vi "Manual Test.vi"() -> ()   [LabVIEW 2018, in "Omega Platinum Series.lvlib"]
uses:
  <instrlib>/Omega Platinum Series/Omega Platinum Series.lvlib
  <instrlib>/Omega Platinum Series/Public/Type Defs/Filter Constant.ctl
  <instrlib>/Omega Platinum Series/Public/Type Defs/Setpoint Type.ctl
  <instrlib>/Omega Platinum Series/Public/Type Defs/Display Temperature Units.ctl
  <instrlib>/Omega Platinum Series/Public/Type Defs/System State.ctl
panel:
  in  "Change Retry Attempts":bool
  in  "Retry Attempts (0)":i32 min=0
  in  "Get Current System State Btn":bool
  out "Current System State":T1
  out "Running":bool
  in  "Start/Stop Btn":bool
  out "Status Setpoint 2 Type":T2=enum."Deviation"
  in  "Change Address Btn":bool
  in  "Initialize Resource Btn":bool
  out "Status Serial Address (hex)":i32 format="%x"
  in  "Get Serial Address Btns":bool
  in  "Get Current Temperature Btn":bool
  out "Current Temperature Reading":string
  in  "Configure Temperature Units":T3
  in  "Set Temperature Units Btn":bool
  in  "Get Temperature Units Btn":bool
  out "Status Temperature Units":string
  in  "Setpoint 2 Type":T2=enum."Deviation"
  in  "Get Setpoint 2 Btn":bool
  in  "Set Setpoint 2 Btn":bool
  out "Status Setpoint 2":dbl
  in  "Configure Setpoint 2":dbl
  in  "Get Setpoint 1 Btn":bool
  in  "Set Setpoint 1 Btn":bool
  out "Status Setpoint 1":dbl
  in  "Configure Setpoint 1":dbl
  in  "Get Filter Constant Btn":bool
  out "Status Filter Constant":T4
  in  "Configure Filter Constant Btn":bool
  in  "Unit ID (-1, 0-199)":i32
  in  "Configure Filter Constant":T4
  out "error out":errorcluster
  in  "stop":bool
  in  "error in (no error)":errorcluster
  in  "Get Firmware Version Btn":bool
  out "Firmware Version":string
  in  "VISA resource name":refnum<visa-resource-name>
  # "Omega Platinum Series"
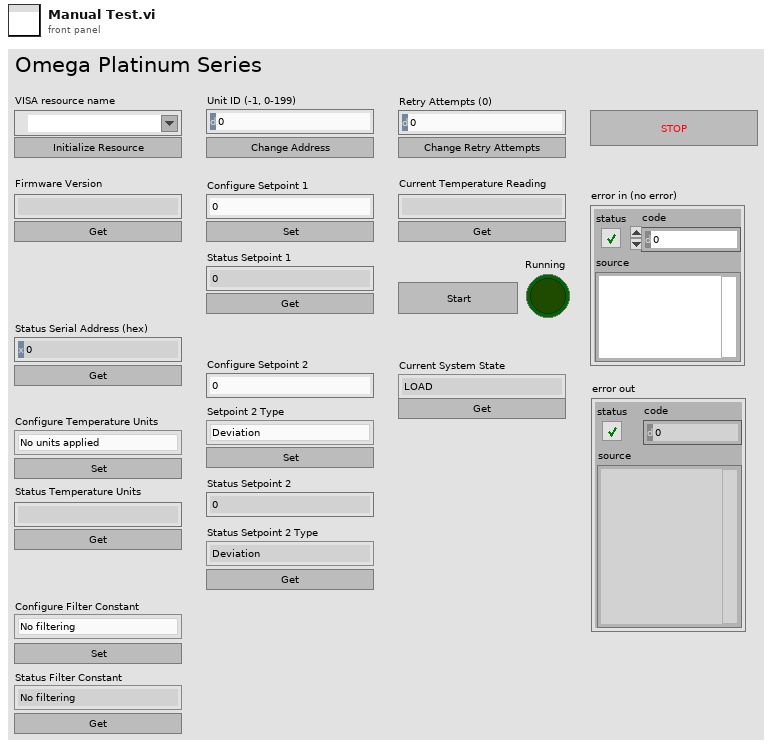
[diagram p1: front panel]
types:
  T1 = typedef "Omega Platinum Series.lvlib/System State.ctl" = enum16{"LOAD", "IDLE", "INPUT_ADJUST", "CONTROL_ADJUST", "MODIFY", "WAIT", "RUN", "STANDBY", "STOP", "PAUSE", "FAULT", "SHUTDOWN", "AUTOTUNE"}
  T2 = typedef "Omega Platinum Series.lvlib/Setpoint Type.ctl" = enum16{"Fixed Constant", "Deviation"}
  T3 = typedef "Omega Platinum Series.lvlib/Display Temperature Units.ctl" = enum16{"No units applied", "Celsius", "Fahrenheit"}
  T4 = typedef "Omega Platinum Series.lvlib/Filter Constant.ctl" = enum16{"No filtering", "X 2 filtering", "X 4 filtering", "X 8 filtering", "X 16 filtering", "X 32 filtering", "X 64 filtering", "X 128 filtering"}
  T5 = cluster{"Baud Rate":u32, "Parity":u16, "Flow Control":u16, "Data Bits":u16, "Stop Bits":u16}
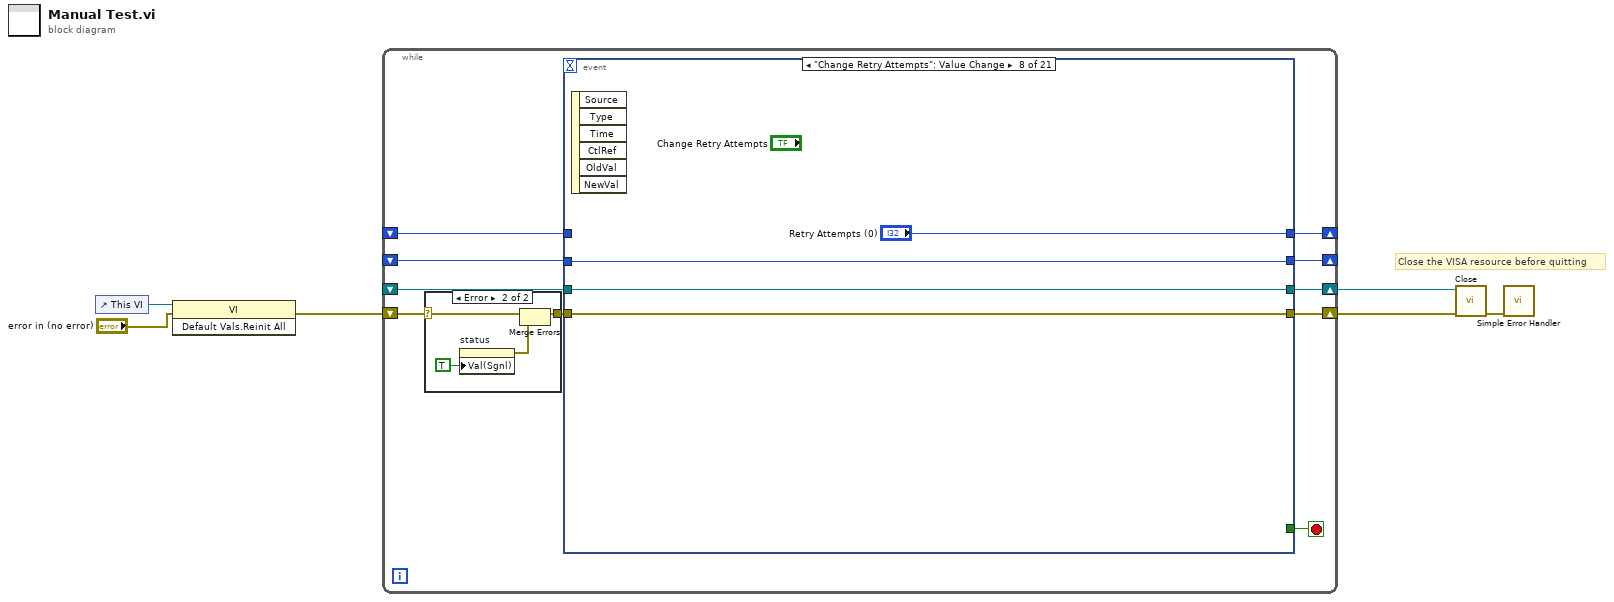
[diagram p0: block diagram]
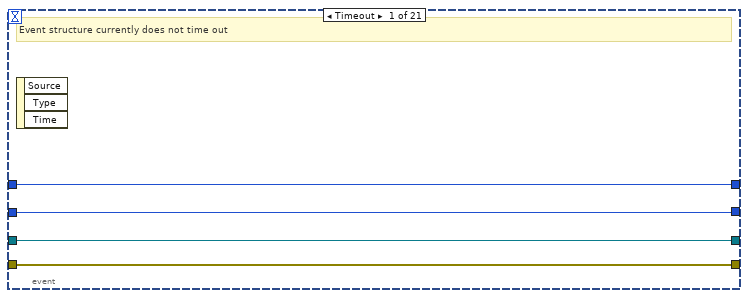
[diagram p3: hidden frame]
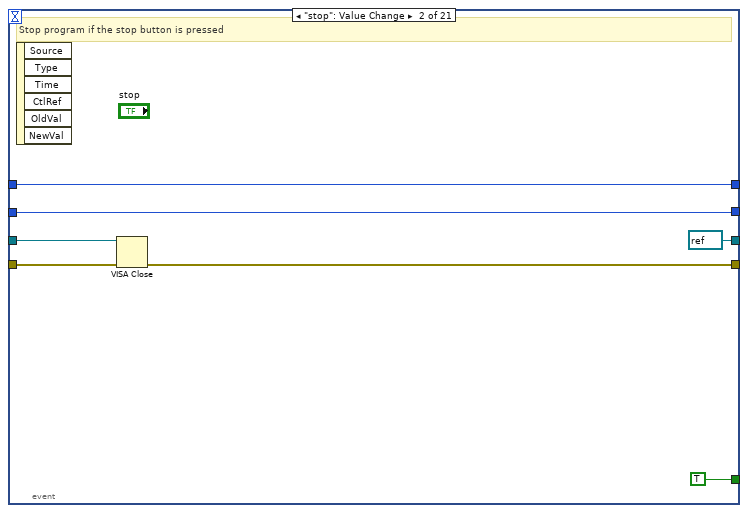
[diagram p4: hidden frame]
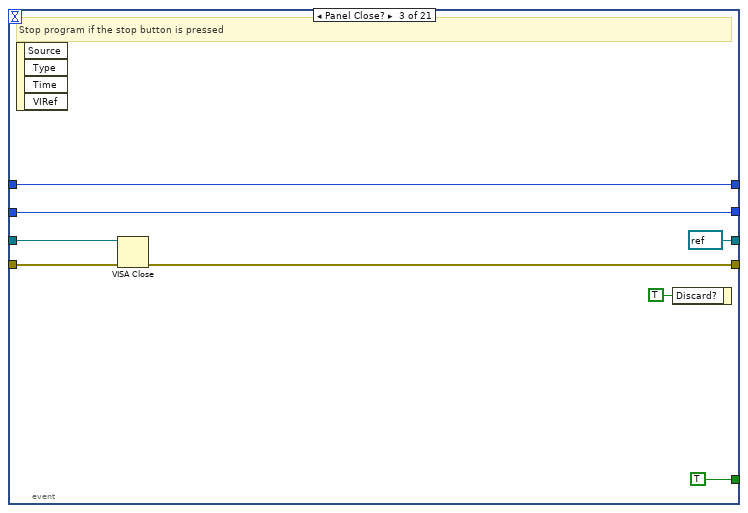
[diagram p5: hidden frame]
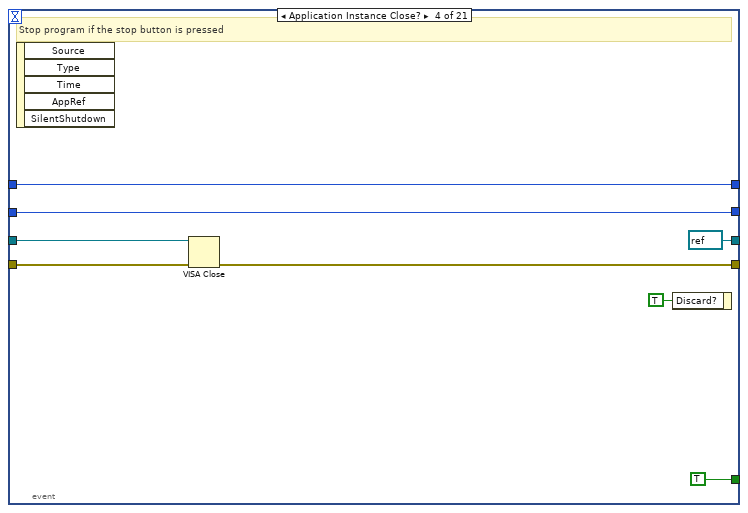
[diagram p6: hidden frame]
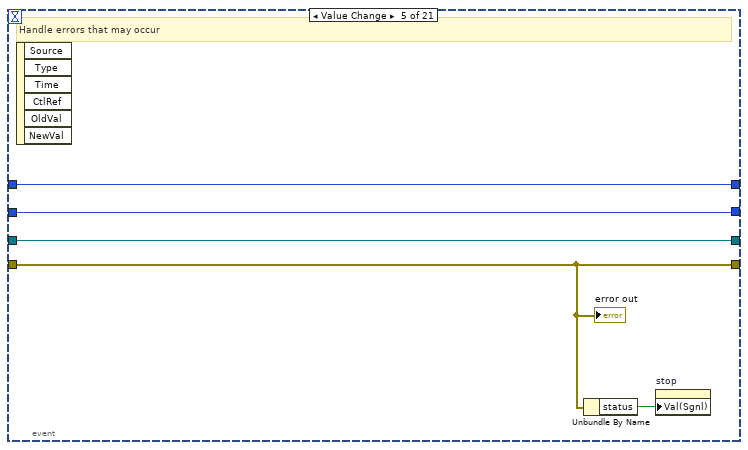
[diagram p7: hidden frame]
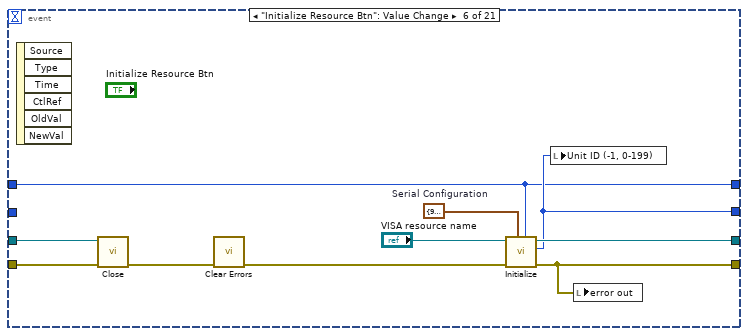
[diagram p8: hidden frame]
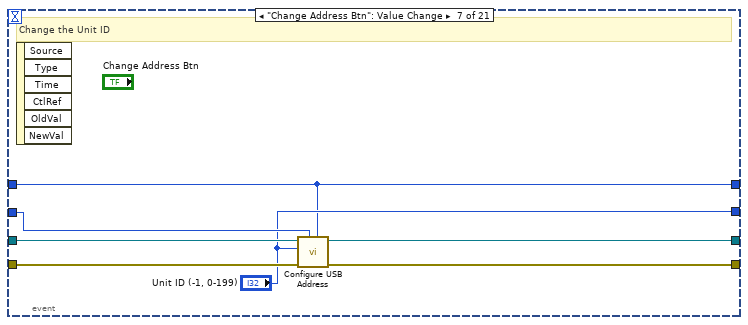
[diagram p9: hidden frame]
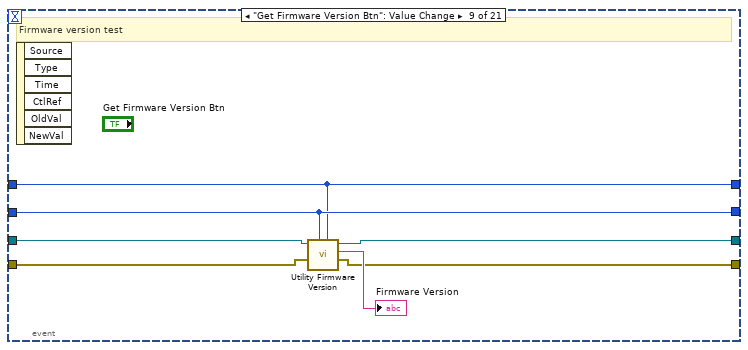
[diagram p10: hidden frame]
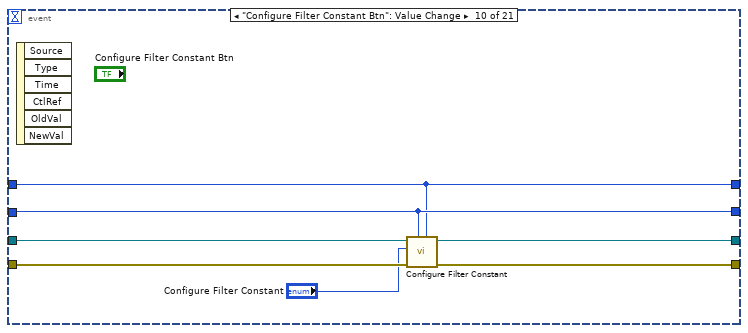
[diagram p11: hidden frame]
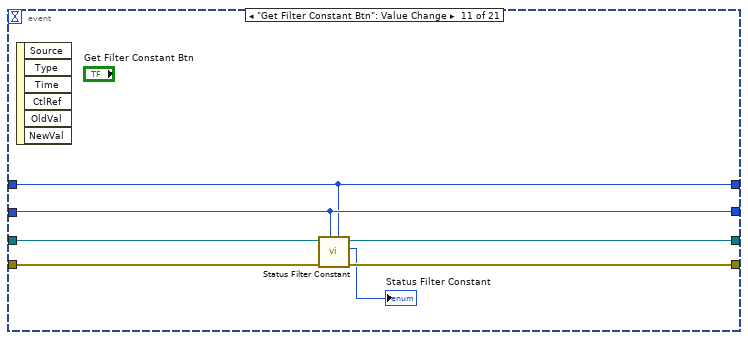
[diagram p12: hidden frame]
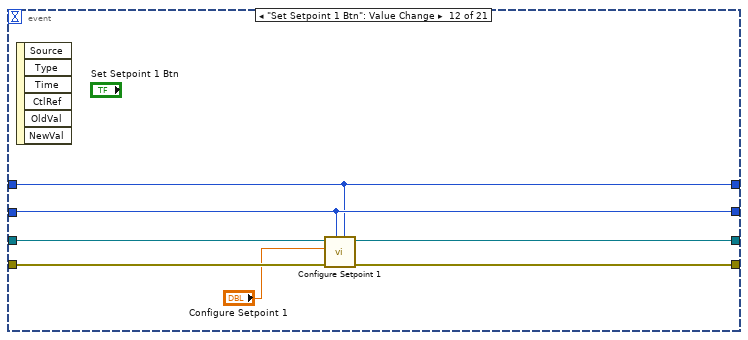
[diagram p13: hidden frame]
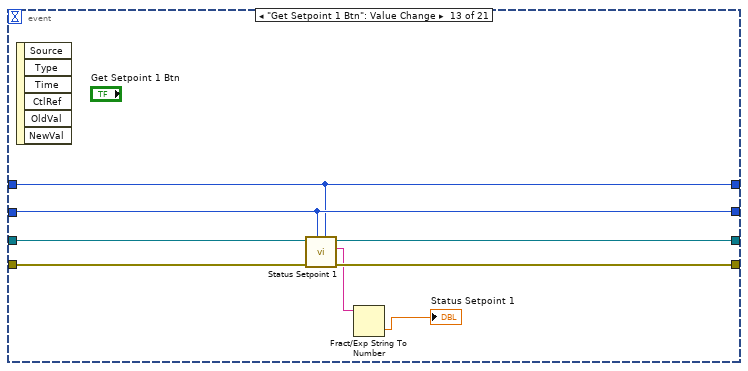
[diagram p14: hidden frame]
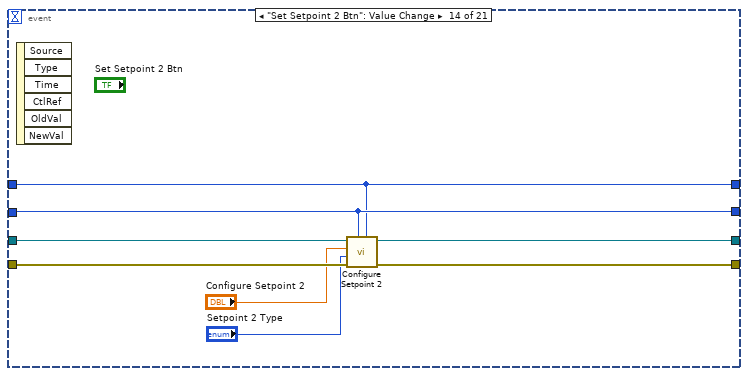
[diagram p15: hidden frame]
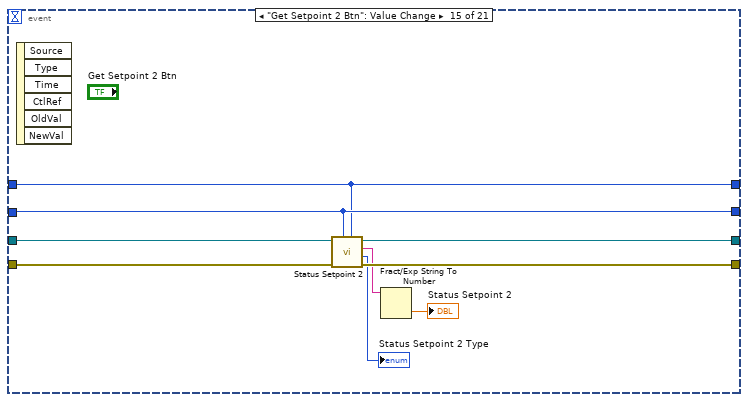
[diagram p16: hidden frame]
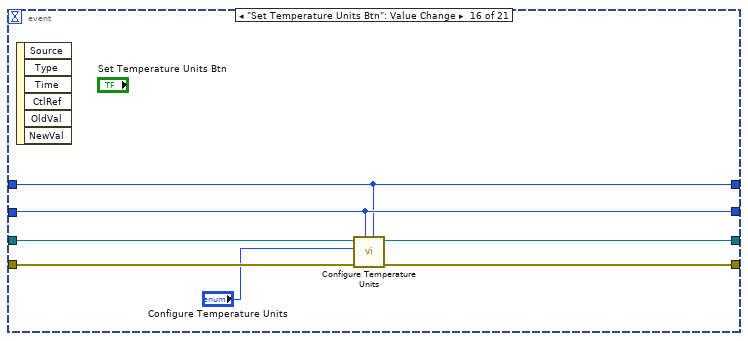
[diagram p17: hidden frame]
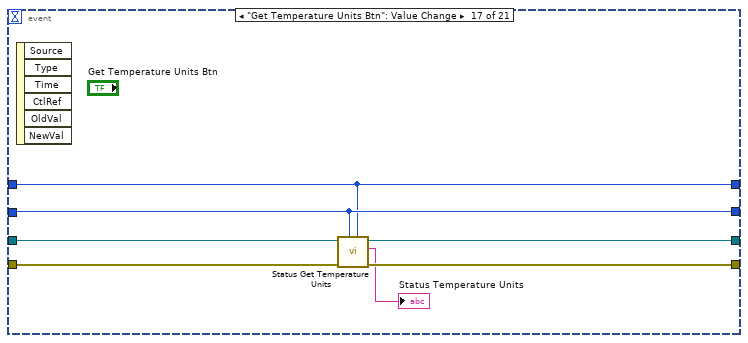
[diagram p18: hidden frame]
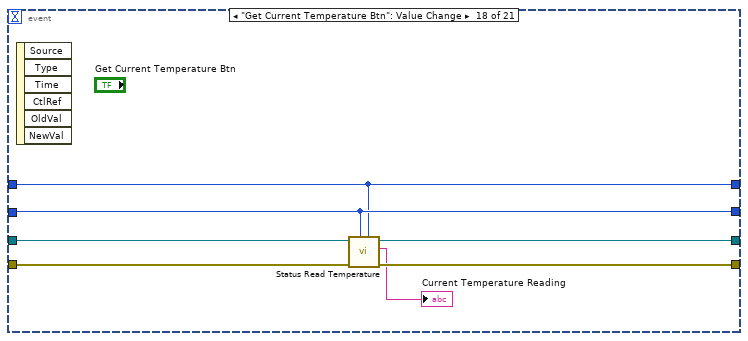
[diagram p19: hidden frame]
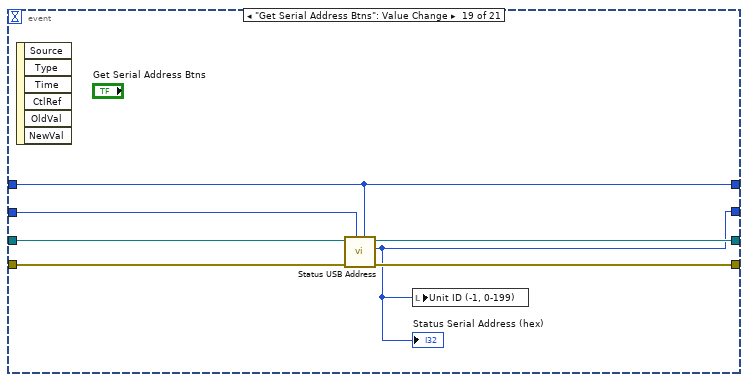
[diagram p20: hidden frame]
diagram:
  # "Close the VISA resource before quitting"
  n1 = control-ref of="This VI"() -> (w4:refnum<vi>)
  n2 = invoke class="VI" method="Default Vals.Reinit All"(reference=w4, error in="error in (no error)") -> (error out=w2:errorcluster)  [unwired: 1 in, 2 out]
  n3 = while {
    shift-right: [w13] -> w5
    shift-left: w2 -> [w12]
    shift-right: [w15] -> w6
    shift-left: _ -> [w16]
    shift-right: [w9] -> _
    shift-left: _ -> [w10]
    shift-right: [w7] -> _
    shift-left: _ -> [w8]
    stop <- w14 stop-if-true
    # "Manual Testing Finite State Machine"
    n4 = case shown="Error" w12 {
      selector: w12 -> [w17 w21]
      tunnel: [w17 w19] -> w11
      frame No Error {
      }
      frame Error {
        n5 = property on="status" class="Bool (strict)"("Val(Sgnl)"=TRUE ("Value (Signaling)")) -> (error out=w18:errorcluster)  [unwired: 2 in, 1 out]
        n6 = Merge Errors(w21, w18) -> (w19:errorcluster)
      }
    }
    n7 = event shown="[7] \"Change Retry Attempts\": Value Change" {
      selector: _ -> [_ _ _ _ _ _ _ _ _ _ _ _ _ _ _ _ _ _ _ _ _]
      dyn-events: _ -> [_ _ _ _ _ _ _ _ _ _ _ _ _ _ _ _ _ _ _ _ _]
      timeout: _ -> [_ _ _ _ _ _ _ _ _ _ _ _ _ _ _ _ _ _ _ _ _]
      tunnel: w16 -> [w25 w31 w35 w43 w53 w58 w70 w72 w80 w88 w94 w101 w109 w117 w126 w133 w140 w147 w155 w162 w183]
      tunnel: [w25 refnum<visa-resource-name> refnum ("VISA resource name (out)") refnum<visa-resource-name> refnum ("VISA resource name (out)") refnum<visa-resource-name> refnum ("VISA resource name (out)") w53 w61 w69 w72 w79 w86 w93 w100 w108 w116 w125 w132 w139 w146 w154 w160 w179] -> w15
      tunnel: w11 -> [w24 w29 w39 w47 w52 w62 w68 w71 w78 w87 w95 w102 w110 w118 w127 w134 w141 w148 w153 w161 w182]
      tunnel: [w24 w28 w36 w44 w52 w57 w67 w71 w77 w85 w92 w99 w107 w115 w124 w131 w138 w145 w152 w159 w181] -> w13
      tunnel: [_ TRUE TRUE TRUE _ _ _ _ _ _ _ _ _ _ _ _ _ _ _ _ _] -> w14
      tunnel: w10 -> [w23 w30 w38 w46 w51 _ w66 w73 w76 w84 w90 w98 w104 w112 w122 w129 w136 w143 w151 w163 w180]
      tunnel: [w23 w30 w38 w46 w51 w56 "Unit ID (-1, 0-199)" w73 w76 w84 w90 w98 w104 w112 w122 w129 w136 w143 w150 w158 w180] -> w9
      tunnel: w8 -> [w22 w26 w33 w41 w49 w54 w64 _ w75 w82 w89 w96 w103 w111 w119 w128 w135 w142 w149 w157 w178]
      tunnel: [w22 w26 w33 w41 w49 w54 w64 "Retry Attempts (0)" w75 w82 w89 w96 w103 w111 w119 w128 w135 w142 w149 w156 w178] -> w7
      event Timeout {
        # "Event structure currently does not time out"
        n8 = event-data() -> ()  [unwired: 1 in, 3 out]
      }
      event "stop": Value Change {
        # "Stop program if the stop button is pressed"
        n9 = event-data() -> ()  [unwired: 1 in, 6 out]
        n10 = VISA Close(VISA resource name=w31, error in (no error)=w29) -> (error out=w28:errorcluster)
      }
      event Panel Close? {
        # "Stop program if the stop button is pressed"
        n11 = event-data() -> ()  [unwired: 1 in, 4 out]
        n12 = VISA Close(VISA resource name=w35, error in (no error)=w39) -> (error out=w36:errorcluster)
        n13 = event-data("Discard?"=TRUE) -> ()  [unwired: 1 in, 1 out]
      }
      event Application Instance Close? {
        # "Stop program if the stop button is pressed"
        n14 = event-data() -> ()  [unwired: 1 in, 5 out]
        n15 = VISA Close(VISA resource name=w43, error in (no error)=w47) -> (error out=w44:errorcluster)
        n16 = event-data("Discard?"=TRUE) -> ()  [unwired: 1 in, 1 out]
      }
      event "error out.status": Value Change {
        # "Handle errors that may occur"
        n17 = event-data() -> ()  [unwired: 1 in, 6 out]
        n18 = Unbundle By Name(w52) -> ("status"=w50:bool)
        n19 = property on="stop" class="Bool (strict)"("Val(Sgnl)"=w50) -> ()  [unwired: 2 in, 2 out]
        "error out" <- w52
      }
      event "Initialize Resource Btn": Value Change {
        w63 = T5 {"Baud Rate"=9600, "Parity"=0, "Flow Control"=0, "Data Bits"=8, "Stop Bits"=10}  # Serial Configuration
        n20 = event-data() -> ()  [unwired: 1 in, 6 out]
        n21 = call <instrlib>:"Close.vi"("error in (no error)"=w62, "VISA resource name"=w58) -> ("error out"=w59:errorcluster)  [unwired: 9 in]
        n22 = call <vilib>:"Clear Errors.vi"("error in (no error)"=w59) -> ("error out"=w55:errorcluster)  [unwired: 5 in, 1 out]
        n23 = call <instrlib>:"Initialize.vi"("Retry Attempts (0)"=w54, "Serial Configuration"=w63, "error in (no error)"=w55, "VISA resource name"="VISA resource name") -> ("error out"=w57:errorcluster, "Address ID (-1 if ID Query = False)"=w56:i32, "VISA resource name out"=w61:refnum<visa-resource-name>)  [unwired: 5 in]
        n24 = local write "Unit ID (-1, 0-199)"(w56) -> ()
        n25 = local write "error out"(w57) -> ()
      }
      event "Change Address Btn": Value Change {
        # "Change the Unit ID"
        n26 = event-data() -> ()  [unwired: 1 in, 6 out]
        n27 = call <instrlib>:"Configure USB Address.vi"("Retry Attempts (0)"=w64, "Current Address (-1)"=w66, "error in (no error)"=w68, "New Address"="Unit ID (-1, 0-199)", "VISA resource name (in)"=w70) -> ("error out"=w67:errorcluster, "VISA resource name (out)"=w69:refnum<visa-resource-name>)  [unwired: 4 in, 1 out]
      }
      event "Change Retry Attempts": Value Change {
        n28 = event-data() -> ()  [unwired: 1 in, 6 out]
      }
      event "Get Firmware Version Btn": Value Change {
        # "Firmware version test"
        n29 = event-data() -> ()  [unwired: 1 in, 6 out]
        n30 = call <instrlib>:"Utility Firmware Version.vi"("Retry Attempts (0)"=w75, "Unit ID (-1)"=w76, "error in"=w78, "VISA resource name"=w80) -> ("error out"=w77:errorcluster, "Firmware Version"=→"Firmware Version":string, "VISA resource name out"=w79:refnum<visa-resource-name>)  [unwired: 5 in]
      }
      event "Configure Filter Constant Btn": Value Change {
        n31 = event-data() -> ()  [unwired: 1 in, 6 out]
        n32 = call <instrlib>:"Configure Filter Constant.vi"("Retry Attempts (0)"=w82, "Unit Address (-1)"=w84, "error in (no error)"=w87, "Filter Constant"="Configure Filter Constant", "VISA resource name (in)"=w88) -> ("error out"=w85:errorcluster, "VISA resource name (out)"=w86:refnum<visa-resource-name>)  [unwired: 4 in, 1 out]
      }
      event "Get Filter Constant Btn": Value Change {
        n33 = event-data() -> ()  [unwired: 1 in, 6 out]
        n34 = call <instrlib>:"Status Filter Constant.vi"("Retry Attempts (0)"=w89, "Unit Address (-1)"=w90, "error in (no error)"=w95, "VISA resource name (in)"=w94) -> ("error out"=w92:errorcluster, "Filter Constant"=→"Status Filter Constant":T4, "VISA resource name (out)"=w93:refnum<visa-resource-name>)  [unwired: 5 in]
      }
      event "Set Setpoint 1 Btn": Value Change {
        n35 = event-data() -> ()  [unwired: 1 in, 6 out]
        n36 = call <instrlib>:"Configure Setpoint 1.vi"("Retry Attempts (0)"=w96, "Unit Address (-1)"=w98, "error in (no error)"=w102, "Setpoint value"="Configure Setpoint 1", "VISA resource name (in)"=w101) -> ("error out"=w99:errorcluster, "VISA resource name (out)"=w100:refnum<visa-resource-name>)  [unwired: 4 in, 1 out]
      }
      event "Get Setpoint 1 Btn": Value Change {
        n37 = event-data() -> ()  [unwired: 1 in, 6 out]
        n38 = call <instrlib>:"Status Setpoint 1.vi"("Retry Attempts (0)"=w103, "Unit Address (-1)"=w104, "error in (no error)"=w110, "VISA resource name (in)"=w109) -> ("error out"=w107:errorcluster, "Setpoint 1"=w106:string, "VISA resource name (out)"=w108:refnum<visa-resource-name>)  [unwired: 5 in]
        n39 = Fract/Exp String To Number(string=w106) -> (number=→"Status Setpoint 1":dbl)  [unwired: 3 in, 1 out]
      }
      event "Set Setpoint 2 Btn": Value Change {
        n40 = event-data() -> ()  [unwired: 1 in, 6 out]
        n41 = call <instrlib>:"Configure Setpoint 2.vi"("Retry Attempts (0)"=w111, "Unit Address (-1)"=w112, "error in (no error)"=w118, "Setpoint Type (deviation)"="Setpoint 2 Type", "Setpoint value"="Configure Setpoint 2", "VISA resource name (in)"=w117) -> ("error out"=w115:errorcluster, "VISA resource name (out)"=w116:refnum<visa-resource-name>)  [unwired: 3 in, 1 out]
      }
      event "Get Setpoint 2 Btn": Value Change {
        n42 = event-data() -> ()  [unwired: 1 in, 6 out]
        n43 = call <instrlib>:"Status Setpoint 2.vi"("Retry Attempts (0)"=w119, "Unit Address (-1)"=w122, "error in (no error)"=w127, "VISA resource name (in)"=w126) -> ("error out"=w124:errorcluster, "Setpoint Type"=→"Status Setpoint 2 Type":T2, "Setpoint 2"=w121:string, "VISA resource name (out)"=w125:refnum<visa-resource-name>)  [unwired: 4 in]
        n44 = Fract/Exp String To Number(string=w121) -> (number=→"Status Setpoint 2":dbl)  [unwired: 3 in, 1 out]
      }
      event "Set Temperature Units Btn": Value Change {
        n45 = event-data() -> ()  [unwired: 1 in, 6 out]
        n46 = call <instrlib>:"Configure Temperature Units.vi"("Retry Attempts (0)"=w128, "Unit Address (-1)"=w129, "error in (no error)"=w134, "Temperature Units (Celsius)"="Configure Temperature Units", "VISA resource name (in)"=w133) -> ("error out"=w131:errorcluster, "VISA resource name (out)"=w132:refnum<visa-resource-name>)  [unwired: 4 in, 1 out]
      }
      event "Get Temperature Units Btn": Value Change {
        n47 = event-data() -> ()  [unwired: 1 in, 6 out]
        n48 = call <instrlib>:"Status Get Temperature Units.vi"("Retry Attempts (0)"=w135, "Unit Address (-1)"=w136, "error in (no error)"=w141, "VISA resource name (in)"=w140) -> ("error out"=w138:errorcluster, "Temperature Units"=→"Status Temperature Units":string, "VISA resource name (out)"=w139:refnum<visa-resource-name>)  [unwired: 5 in]
      }
      event "Get Current Temperature Btn": Value Change {
        n49 = event-data() -> ()  [unwired: 1 in, 6 out]
        n50 = call <instrlib>:"Status Read Temperature.vi"("Retry Attempts (0)"=w142, "Unit Address (-1)"=w143, "error in (no error)"=w148, "VISA resource name (in)"=w147) -> ("error out"=w145:errorcluster, "Temperature"=→"Current Temperature Reading":string, "VISA resource name (out)"=w146:refnum<visa-resource-name>)  [unwired: 5 in]
      }
      event "Get Serial Address Btns": Value Change {
        n51 = event-data() -> ()  [unwired: 1 in, 6 out]
        n52 = call <instrlib>:"Status USB Address.vi"("Retry Attempts (0)"=w149, "Unit Address (-1)"=w151, "error in (no error)"=w153, "VISA resource name (in)"=w155) -> ("error out"=w152:errorcluster, "Address"=w150:i32, "VISA resource name (out)"=w154:refnum<visa-resource-name>)  [unwired: 5 in]
        "Status Serial Address (hex)" <- w150
        n53 = local write "Unit ID (-1, 0-199)"(w150) -> ()
      }
      event "Start/Stop Btn": Value Change {
        n54 = event-data() -> ("NewVal"=→"Running":bool)  [unwired: 1 in, 5 out]
        n55 = case shown="True" "Start/Stop Btn" {
          tunnel: w163 -> [w167 w173]
          tunnel: w162 -> [w171 w177]
          tunnel: w161 -> [w169 w175]
          tunnel: [w170 w176] -> w160
          tunnel: [w168 w174] -> w159
          tunnel: [w167 w173] -> w158
          tunnel: w157 -> [w166 w172]
          tunnel: [w166 w172] -> w156
          frame False {
            # "Stop the controller."
            n56 = call <instrlib>:"Action Stop.vi"("Retry Attempts (0)"=w166, "Unit Address (-1)"=w167, "error in (no error)"=w169, "VISA resource name (in)"=w171) -> ("error out"=w168:errorcluster, "VISA resource name (out)"=w170:refnum<visa-resource-name>)  [unwired: 5 in, 1 out]
          }
          frame True {
            # "Start the controller."
            n57 = call <instrlib>:"Action Run.vi"("Retry Attempts (0)"=w172, "Unit Address (-1)"=w173, "error in (no error)"=w175, "VISA resource name (in)"=w177) -> ("error out"=w174:errorcluster, "VISA resource name (out)"=w176:refnum<visa-resource-name>)  [unwired: 5 in, 1 out]
          }
        }
      }
      event "Get Current System State Btn": Value Change {
        n58 = event-data() -> ()  [unwired: 1 in, 6 out]
        n59 = call <instrlib>:"Status System State.vi"("Retry Attempts (0)"=w178, "Unit Address (-1)"=w180, "error in (no error)"=w182, "VISA resource name (in)"=w183) -> ("error out"=w181:errorcluster, "System State"=→"Current System State":T1, "VISA resource name (out)"=w179:refnum<visa-resource-name>)  [unwired: 5 in]
      }
    }
  }
  n60 = call <instrlib>:"Close.vi"("error in (no error)"=w5, "VISA resource name"=w6) -> ("error out"=w1:errorcluster)  [unwired: 9 in]
  n61 = call <vilib>:"Simple Error Handler.vi"("error in (no error)"=w1) -> ()  [unwired: 4 in, 5 out]
